vi "NOPTR_Mem_DataToU8Array.vi"(8 "error in (no error)":errorcluster, 10 "Payload":variant, 11 "AddrQueueIn":refnum<queue>) -> (0 "error out":errorcluster, 1 "Supported Type?":bool, 2 "ByteArray":u8[](array[numeric]), 3 "AddrQueueOut":refnum<queue>)   [LabVIEW 2019, in "Memory Data Access.lvlib"]
uses:
  Memory Data Access.lvlib
  <vilib>/Utility/Data Type/Type Definitions/Data Type.ctl
  Global/Global.vi
  <vilib>/Utility/Data Type/NI_Data Type.lvlib
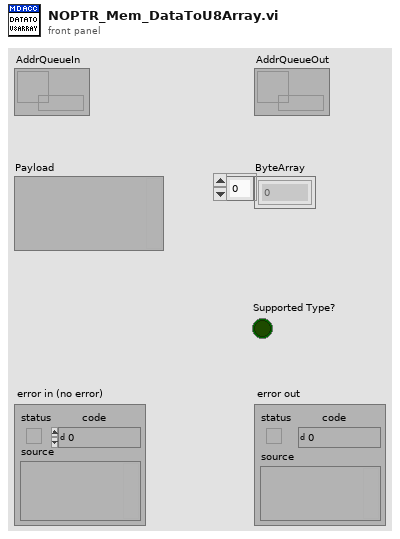
[diagram p1: front panel]
types:
  T1 = typedef "NI_Data Type.lvlib/Data Type.ctl" = enum8{"Invalid Type", "Void", "I8", "I16", "I32", "I64", "U8", "U16", "U32", "U64", "Single Float", "Double Float", "Extended Float", "Single Complex", "Double Complex", "Extended Complex", "Enum U8", "Enum U16", "Enum U32", "Enum U64", "Single Float With Unit", "Double Float With Unit", "Extended Float With Unit", "Single Complex with Unit", "Double Complex with Unit", "Extended Complex with Unit", "Boolean", "String", "Path", "Picture", "Tag", "Array", "Cluster", "Variant", "LV Variant", "Waveform", "Timestamp", "Digital Waveform", "Digital Data", "ExpressData", "Refnum", "External Data", "VI", "Poly VI", "LabVIEW Class Instance", "Fixed Point", "Set Collection", "Map Collection"}
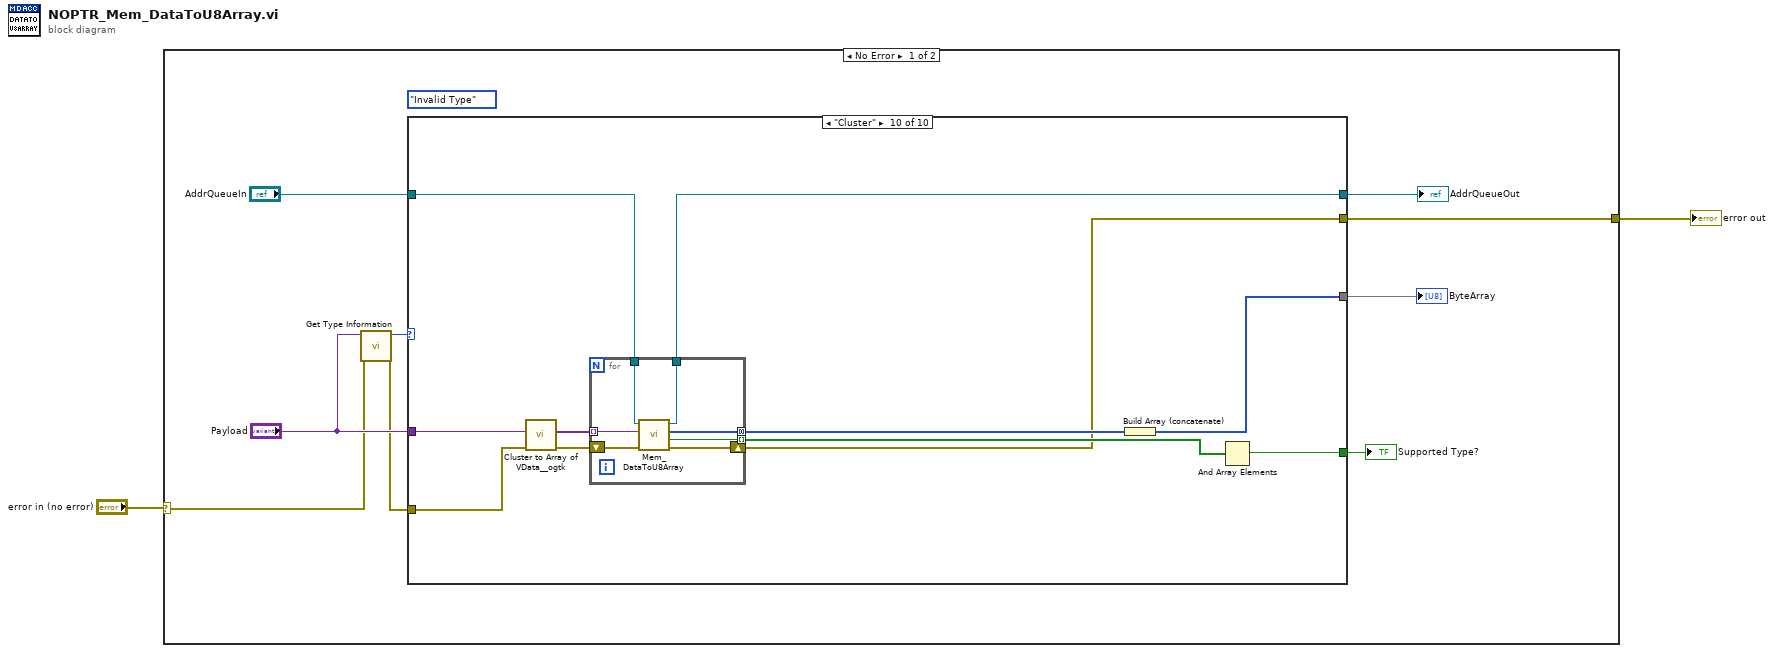
[diagram p0: block diagram]
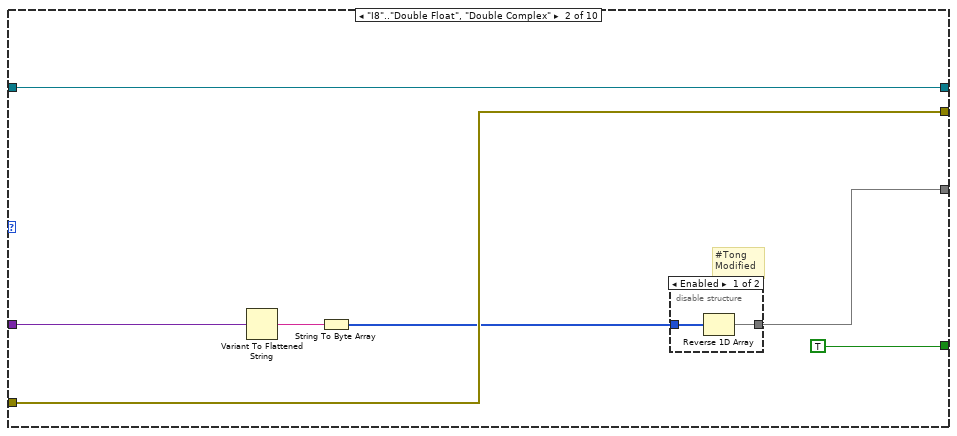
[diagram p3: hidden frame]
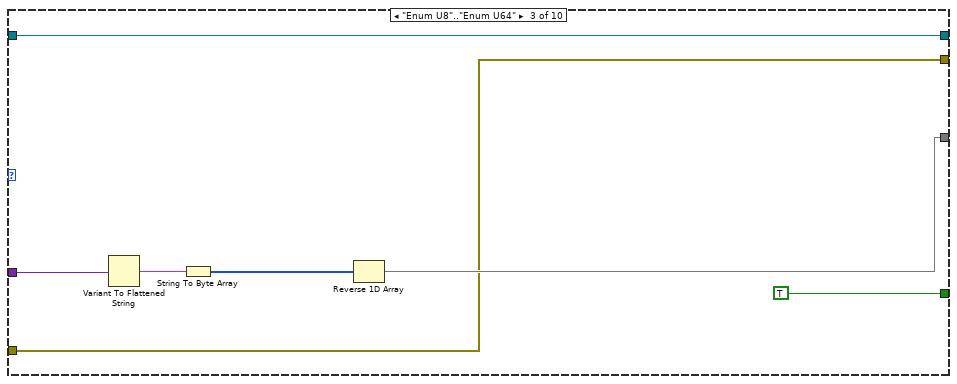
[diagram p5: hidden frame]
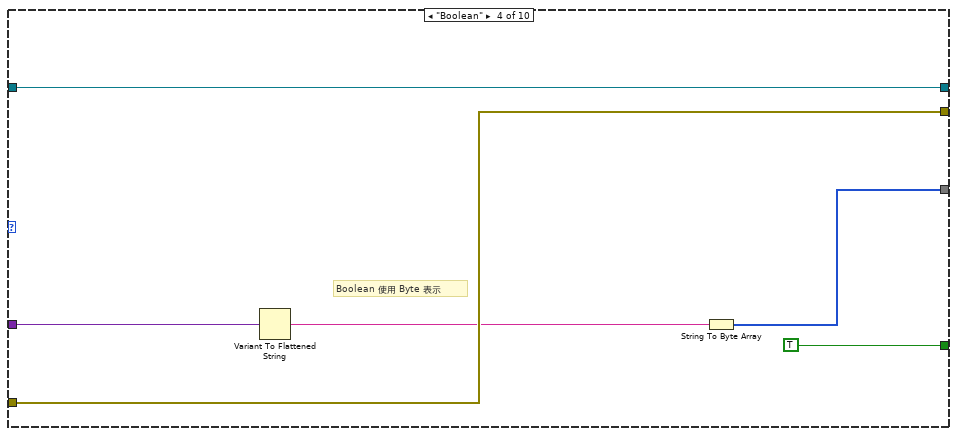
[diagram p6: hidden frame]
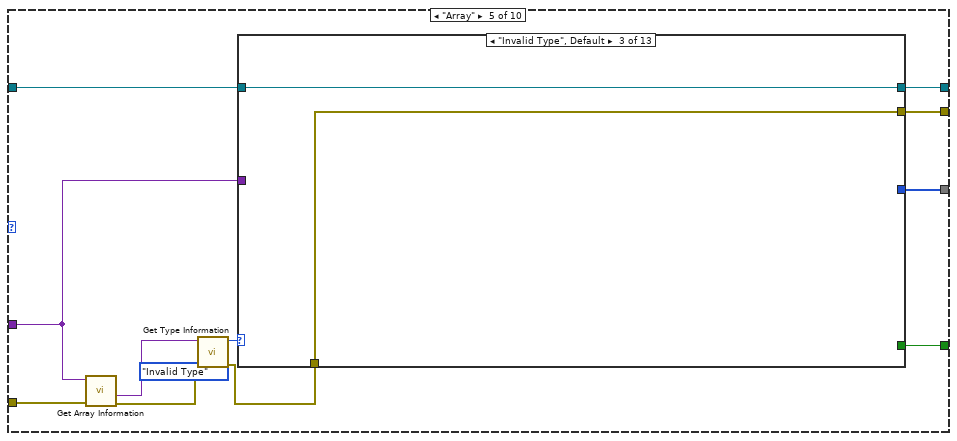
[diagram p7: hidden frame]
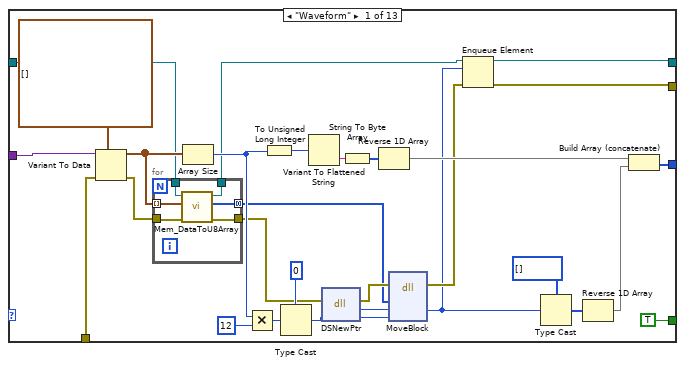
[diagram p8: hidden frame]
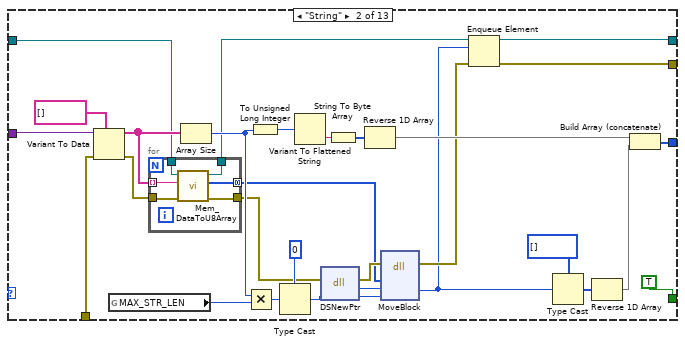
[diagram p9: hidden frame]
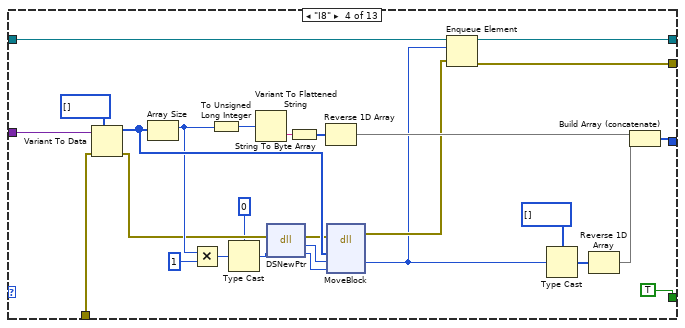
[diagram p10: hidden frame]
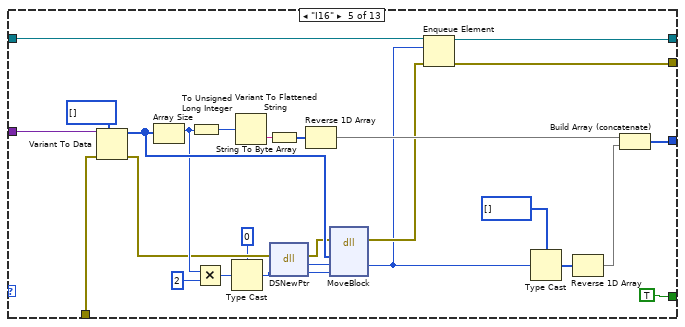
[diagram p11: hidden frame]
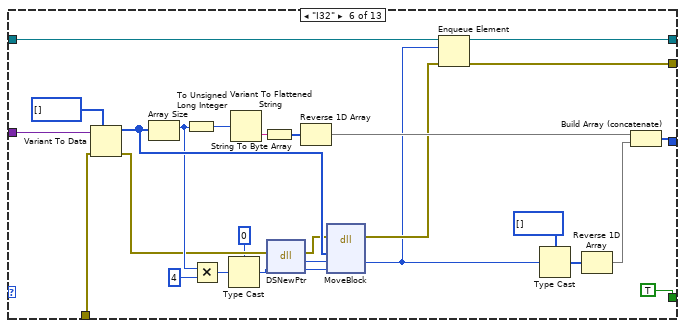
[diagram p12: hidden frame]
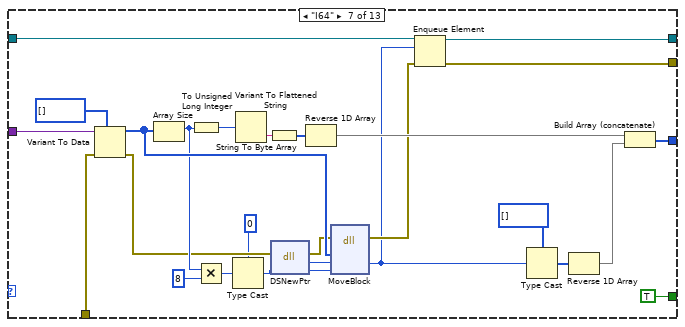
[diagram p13: hidden frame]
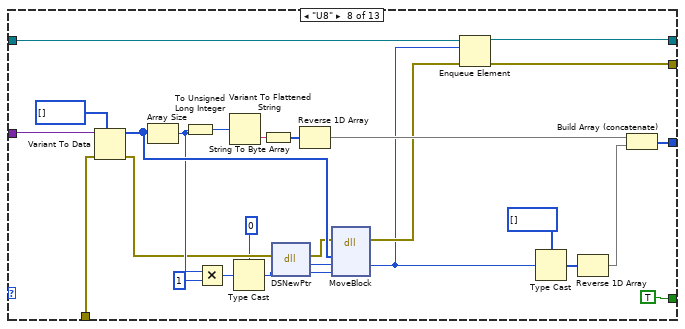
[diagram p14: hidden frame]
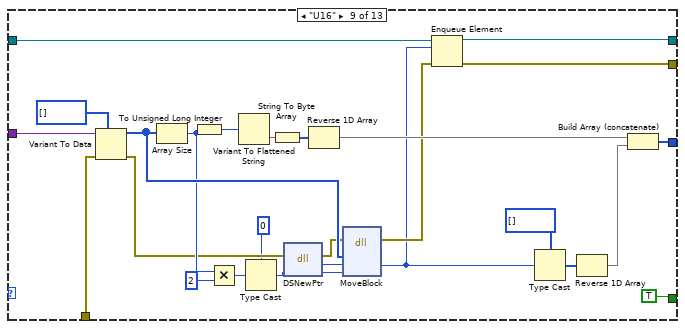
[diagram p15: hidden frame]
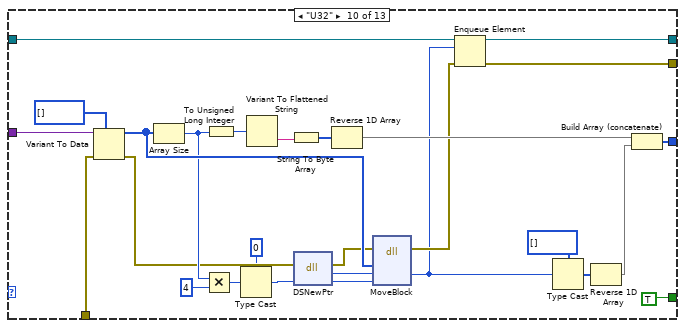
[diagram p16: hidden frame]
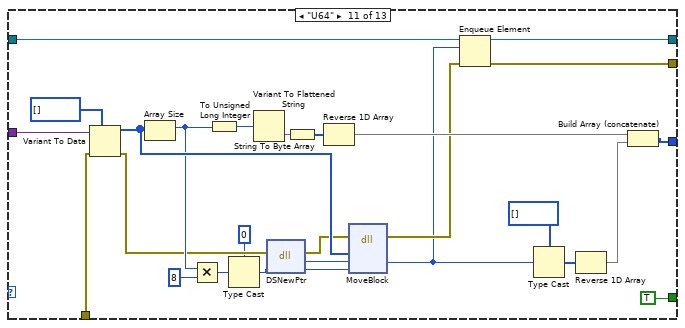
[diagram p17: hidden frame]
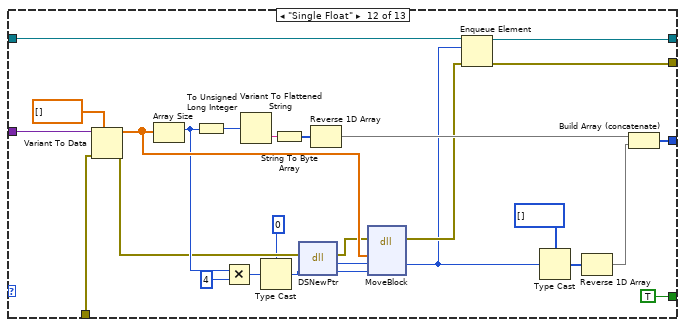
[diagram p18: hidden frame]
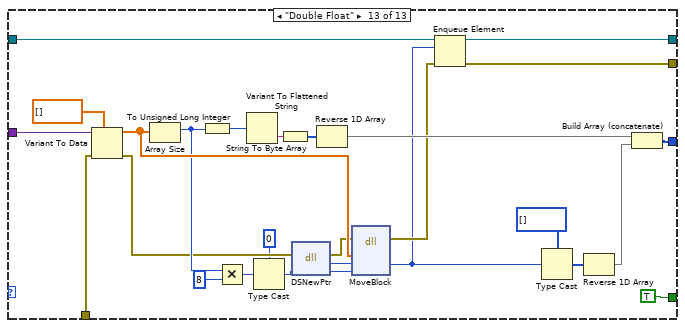
[diagram p19: hidden frame]
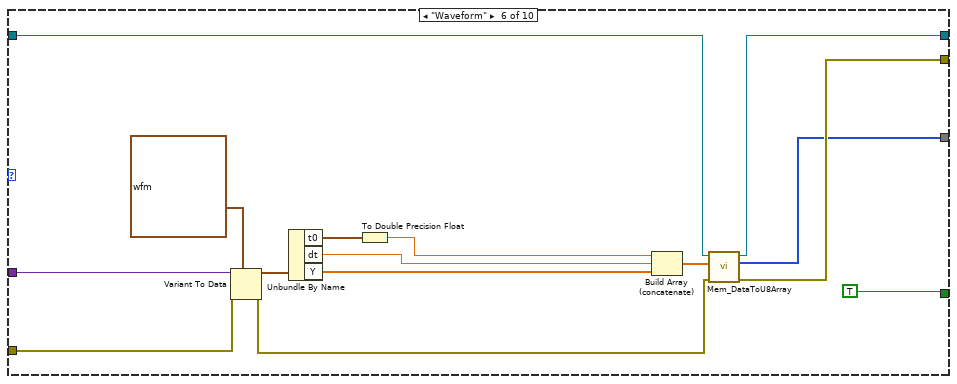
[diagram p20: hidden frame]
diagram:
  n1 = case shown="No Error" "error in (no error)" {
    selector: "error in (no error)" -> [w3 w466]
    tunnel: [w11 w466] -> w2
    frame No Error {
      (unwired) Data_Type."Invalid Type" ("Type")
      n2 = call <vilib>:"Get Type Information.vi"("error in (no error)"=w3, "variant"="Payload") -> ("error out"=w6:errorcluster, "type"=w7:T1)  [unwired: 5 in, 3 out]
      n3 = case shown="\"Cluster\"" w7 {
        tunnel: w6 -> [w13 w20 w26 w36 w44 w398 w409 w429 w438 w450]
        tunnel: [w13 w20 w26 w36 w46 w395 w410 w430 w439 w451] -> w11
        tunnel: [_ w15 w27 w32 w47 w394 w412 w425 w441 w455] -> w10
        tunnel: "Payload" -> [_ w18 w29 w34 w45 w405 w413 w433 w442 w458]
        tunnel: [_ TRUE TRUE ("Supported Type?") TRUE w37 TRUE TRUE TRUE TRUE w453] -> w9
        tunnel: "AddrQueueIn" -> [w12 w14 w24 w31 w40 w393 w407 w424 w435 w449]
        tunnel: [w12 w14 w24 w31 w39 w392 w407 w424 w435 w448] -> w4
        frame "Invalid Type", Default {
        }
        frame "I8".."Double Float", "Double Complex" {
          # "#Tong\nModified"
          n4 = Variant To Flattened String(Variant=w18) -> (data string=w17:string)  [unwired: 1 out]
          n5 = String To Byte Array(string=w17) -> (unsigned byte array=w16:u8[])
          n6 = disable-structure shown="Enabled" {
            disable-tunnel: w16 -> [w22 w23]
            disable-tunnel: [w21 w23] -> w15
            frame Enabled {
              n7 = Reverse 1D Array(array=w22) -> (reversed array=w21:u8[])
            }
            frame Disabled {
            }
          }
        }
        frame "Enum U8".."Enum U64" {
          n8 = Variant To Flattened String(Variant=w29) -> (data string=w30:string)  [unwired: 1 out]
          n9 = String To Byte Array(string=w30) -> (unsigned byte array=w28:u8[])
          n10 = Reverse 1D Array(array=w28) -> (reversed array=w27:u8[])
        }
        frame "Boolean" {
          # "Boolean 使用 Byte 表示"
          n11 = Variant To Flattened String(Variant=w34) -> (data string=w33:string)  [unwired: 1 out]
          n12 = String To Byte Array(string=w33) -> (unsigned byte array=w32:u8[])
        }
        frame "Array" {
          (unwired) Data_Type."Invalid Type" ("type")
          n13 = call <vilib>:"Get Array Information.vi"("error in (no error)"=w44, "variant"=w45) -> ("error out"=w38:errorcluster, "array element data type"=w42:variant)  [unwired: 6 in, 2 out]
          n14 = call <vilib>:"Get Type Information.vi"("error in (no error)"=w38, "variant"=w42) -> ("error out"=w41:errorcluster, "type"=w43:T1)  [unwired: 5 in, 3 out]
          n15 = case shown="\"Invalid Type\", Default" w43 {
            tunnel: [w58 w97 _ w128 w156 w183 w210 w236 w263 w290 w317 w344 w371] -> w47
            tunnel: w45 -> [w57 w98 _ w130 w157 w184 w211 w238 w265 w293 w319 w346 w373]
            tunnel: w41 -> [w56 w96 w120 w129 w155 w182 w209 w237 w264 w292 w318 w345 w372]
            tunnel: [w51 w88 w120 w124 w152 w178 w204 w231 w259 w287 w313 w340 w368] -> w46
            tunnel: w40 -> [w50 w87 w121 w127 w154 w181 w208 w235 w262 w289 w316 w343 w370]
            tunnel: [w55 w90 w121 w126 w153 w180 w207 w234 w261 w285 w315 w342 w367] -> w39
            tunnel: [TRUE ("Supported Type?") TRUE ("Supported Type?") _ TRUE ("Supported Type?") TRUE ("Supported Type?") TRUE ("Supported Type?") TRUE ("Supported Type?") TRUE ("Supported Type?") TRUE ("Supported Type?") TRUE ("Supported Type?") TRUE ("Supported Type?") TRUE ("Supported Type?") TRUE ("Supported Type?")] -> w37
            frame "Waveform" {
              n16 = Variant To Data(error in=w56, type=waveform(dbl)[] [], Variant=w57) -> (data=w62:waveform(dbl)[], error out=w61:errorcluster)
              n17 = for {
                tunnel: w62 -> [w83] mode=indexing
                tunnel: w61 -> [w82]
                tunnel: [w81] -> w59 mode=concatenating
                tunnel: [w80] -> w60
                tunnel: w50 -> [w79]
                tunnel: [w78] -> w49
                n18 = call "Mem_DataToU8Array.vi"("error in (no error)"=w82, "Payload"=w83, "AddrQueueIn"=w79) -> ("error out"=w80:errorcluster, "ByteArray"=w81:u8[], "AddrQueueOut"=w78:refnum<queue>)  [unwired: 5 in, 1 out]
              }
              n19 = Array Size(array=w62) -> (size(s)=w73:i32)
              n20 = Multiply(x=w73, y=12) -> (x*y=w74:i32)
              n21 = To Unsigned Long Integer(number=w73) -> (unsigned 32bit integer=w70:u32)
              n22 = Type Cast(type=u32 0, x=w74) -> (*(type *) &x=w75:u32)
              n23 = Variant To Flattened String(Variant=w70) -> (data string=w69:string)  [unwired: 1 out]
              n24 = dll-call lib="LabVIEW" fn="DSNewPtr"(error in=w60, "size"=w75) -> (error out=w66:errorcluster, "return type"=w76:u64, "size"=w77:u32)  [unwired: 2 in, 1 out]
              n25 = String To Byte Array(string=w69) -> (unsigned byte array=w71:u8[])
              n26 = Reverse 1D Array(array=w71) -> (reversed array=w72:u8[])
              n27 = dll-call lib="LabVIEW" fn="MoveBlock"(error in=w66, "PointerSRC"=w59, "PointerDEST"=w76, "size"=w77) -> (error out=w53:errorcluster, "PointerDEST"=w52:u64)  [unwired: 5 in, 1 out]
              n28 = Enqueue Element(queue=w49, element=w52, error in (no error)=w53) -> (queue out=w55:refnum<queue>, error out=w51:errorcluster)  [unwired: 1 in, 1 out]
              n29 = Type Cast(type=u8[] [], x=w52) -> (*(type *) &x=w68:u8[])
              n30 = Reverse 1D Array(array=w68) -> (reversed array=w67:u8[])
              n31 = Build Array (concatenate)(w72, w67) -> (w58:u8[])
            }
            frame "String" {
              n32 = Variant To Data(error in=w96, type=string[] [], Variant=w98) -> (data=w95:string[], error out=w94:errorcluster)
              n33 = global read "Global.vi" "MAX_STR_LEN"() -> (w91:u32)
              n34 = for {
                tunnel: w95 -> [w119] mode=indexing
                tunnel: w94 -> [w118]
                tunnel: [w117] -> w92 mode=concatenating
                tunnel: [w116] -> w93
                tunnel: w87 -> [w115]
                tunnel: [w114] -> w85
                n35 = call "Mem_DataToU8Array.vi"("error in (no error)"=w118, "Payload"=w119, "AddrQueueIn"=w115) -> ("error out"=w116:errorcluster, "ByteArray"=w117:u8[], "AddrQueueOut"=w114:refnum<queue>)  [unwired: 5 in, 1 out]
              }
              n36 = Array Size(array=w95) -> (size(s)=w109:i32)
              n37 = Multiply(x=w109, y=w91) -> (x*y=w110:u32)
              n38 = To Unsigned Long Integer(number=w109) -> (unsigned 32bit integer=w106:u32)
              n39 = Type Cast(type=u32 0, x=w110) -> (*(type *) &x=w111:u32)
              n40 = Variant To Flattened String(Variant=w106) -> (data string=w105:string)  [unwired: 1 out]
              n41 = dll-call lib="LabVIEW" fn="DSNewPtr"(error in=w93, "size"=w111) -> (error out=w102:errorcluster, "return type"=w112:u64, "size"=w113:u32)  [unwired: 2 in, 1 out]
              n42 = String To Byte Array(string=w105) -> (unsigned byte array=w107:u8[])
              n43 = Reverse 1D Array(array=w107) -> (reversed array=w108:u8[])
              n44 = dll-call lib="LabVIEW" fn="MoveBlock"(error in=w102, "PointerSRC"=w92, "PointerDEST"=w112, "size"=w113) -> (error out=w89:errorcluster, "PointerDEST"=w86:u64)  [unwired: 5 in, 1 out]
              n45 = Enqueue Element(queue=w85, element=w86, error in (no error)=w89) -> (queue out=w90:refnum<queue>, error out=w88:errorcluster)  [unwired: 1 in, 1 out]
              n46 = Type Cast(type=u8[] [], x=w86) -> (*(type *) &x=w104:u8[])
              n47 = Reverse 1D Array(array=w104) -> (reversed array=w103:u8[])
              n48 = Build Array (concatenate)(w108, w103) -> (w97:u8[])
            }
            frame "Invalid Type", Default {
            }
            frame "I8" {
              n49 = Variant To Data(error in=w129, type=i8[] [], Variant=w130) -> (data=w146:i8[], error out=w138:errorcluster)
              n50 = Array Size(array=w146) -> (size(s)=w143:i32)
              n51 = Multiply(x=w143, y=1) -> (x*y=w144:i32)
              n52 = To Unsigned Long Integer(number=w143) -> (unsigned 32bit integer=w140:u32)
              n53 = Type Cast(type=u32 0, x=w144) -> (*(type *) &x=w145:u32)
              n54 = Variant To Flattened String(Variant=w140) -> (data string=w139:string)  [unwired: 1 out]
              n55 = dll-call lib="LabVIEW" fn="DSNewPtr"(error in=w138, "size"=w145) -> (error out=w135:errorcluster, "return type"=w147:u64, "size"=w148:u32)  [unwired: 2 in, 1 out]
              n56 = String To Byte Array(string=w139) -> (unsigned byte array=w141:u8[])
              n57 = Reverse 1D Array(array=w141) -> (reversed array=w142:u8[])
              n58 = dll-call lib="LabVIEW" fn="MoveBlock"(error in=w135, "PointerSRC"=w146, "PointerDEST"=w147, "size"=w148) -> (error out=w125:errorcluster, "PointerDEST"=w123:u64)  [unwired: 5 in, 1 out]
              n59 = Enqueue Element(queue=w127, element=w123, error in (no error)=w125) -> (queue out=w126:refnum<queue>, error out=w124:errorcluster)  [unwired: 1 in, 1 out]
              n60 = Type Cast(type=u8[] [], x=w123) -> (*(type *) &x=w137:u8[])
              n61 = Reverse 1D Array(array=w137) -> (reversed array=w136:u8[])
              n62 = Build Array (concatenate)(w142, w136) -> (w128:u8[])
            }
            frame "I16" {
              n63 = Variant To Data(error in=w155, type=i16[] [], Variant=w157) -> (data=w173:i16[], error out=w165:errorcluster)
              n64 = Array Size(array=w173) -> (size(s)=w170:i32)
              n65 = To Unsigned Long Integer(number=w170) -> (unsigned 32bit integer=w167:u32)
              n66 = Multiply(x=w170, y=2) -> (x*y=w171:i32)
              n67 = Type Cast(type=u32 0, x=w171) -> (*(type *) &x=w172:u32)
              n68 = Variant To Flattened String(Variant=w167) -> (data string=w166:string)  [unwired: 1 out]
              n69 = String To Byte Array(string=w166) -> (unsigned byte array=w168:u8[])
              n70 = dll-call lib="LabVIEW" fn="DSNewPtr"(error in=w165, "size"=w172) -> (error out=w162:errorcluster, "return type"=w174:u64, "size"=w175:u32)  [unwired: 2 in, 1 out]
              n71 = Reverse 1D Array(array=w168) -> (reversed array=w169:u8[])
              n72 = dll-call lib="LabVIEW" fn="MoveBlock"(error in=w162, "PointerSRC"=w173, "PointerDEST"=w174, "size"=w175) -> (error out=w151:errorcluster, "PointerDEST"=w150:u64)  [unwired: 5 in, 1 out]
              n73 = Enqueue Element(queue=w154, element=w150, error in (no error)=w151) -> (queue out=w153:refnum<queue>, error out=w152:errorcluster)  [unwired: 1 in, 1 out]
              n74 = Type Cast(type=u8[] [], x=w150) -> (*(type *) &x=w164:u8[])
              n75 = Reverse 1D Array(array=w164) -> (reversed array=w163:u8[])
              n76 = Build Array (concatenate)(w169, w163) -> (w156:u8[])
            }
            frame "I32" {
              n77 = Variant To Data(error in=w182, type=i32[] [], Variant=w184) -> (data=w200:i32[], error out=w192:errorcluster)
              n78 = Array Size(array=w200) -> (size(s)=w197:i32)
              n79 = To Unsigned Long Integer(number=w197) -> (unsigned 32bit integer=w194:u32)
              n80 = Multiply(x=w197, y=4) -> (x*y=w198:i32)
              n81 = Type Cast(type=u32 0, x=w198) -> (*(type *) &x=w199:u32)
              n82 = Variant To Flattened String(Variant=w194) -> (data string=w193:string)  [unwired: 1 out]
              n83 = String To Byte Array(string=w193) -> (unsigned byte array=w195:u8[])
              n84 = dll-call lib="LabVIEW" fn="DSNewPtr"(error in=w192, "size"=w199) -> (error out=w189:errorcluster, "return type"=w201:u64, "size"=w202:u32)  [unwired: 2 in, 1 out]
              n85 = Reverse 1D Array(array=w195) -> (reversed array=w196:u8[])
              n86 = dll-call lib="LabVIEW" fn="MoveBlock"(error in=w189, "PointerSRC"=w200, "PointerDEST"=w201, "size"=w202) -> (error out=w179:errorcluster, "PointerDEST"=w177:u64)  [unwired: 5 in, 1 out]
              n87 = Enqueue Element(queue=w181, element=w177, error in (no error)=w179) -> (queue out=w180:refnum<queue>, error out=w178:errorcluster)  [unwired: 1 in, 1 out]
              n88 = Type Cast(type=u8[] [], x=w177) -> (*(type *) &x=w191:u8[])
              n89 = Reverse 1D Array(array=w191) -> (reversed array=w190:u8[])
              n90 = Build Array (concatenate)(w196, w190) -> (w183:u8[])
            }
            frame "I64" {
              n91 = Variant To Data(error in=w209, type=i64[] [], Variant=w211) -> (data=w227:i64[], error out=w219:errorcluster)
              n92 = Array Size(array=w227) -> (size(s)=w224:i32)
              n93 = To Unsigned Long Integer(number=w224) -> (unsigned 32bit integer=w221:u32)
              n94 = Multiply(x=w224, y=8) -> (x*y=w225:i32)
              n95 = Type Cast(type=u32 0, x=w225) -> (*(type *) &x=w226:u32)
              n96 = Variant To Flattened String(Variant=w221) -> (data string=w220:string)  [unwired: 1 out]
              n97 = String To Byte Array(string=w220) -> (unsigned byte array=w222:u8[])
              n98 = dll-call lib="LabVIEW" fn="DSNewPtr"(error in=w219, "size"=w226) -> (error out=w216:errorcluster, "return type"=w228:u64, "size"=w229:u32)  [unwired: 2 in, 1 out]
              n99 = Reverse 1D Array(array=w222) -> (reversed array=w223:u8[])
              n100 = dll-call lib="LabVIEW" fn="MoveBlock"(error in=w216, "PointerSRC"=w227, "PointerDEST"=w228, "size"=w229) -> (error out=w206:errorcluster, "PointerDEST"=w205:u64)  [unwired: 5 in, 1 out]
              n101 = Enqueue Element(queue=w208, element=w205, error in (no error)=w206) -> (queue out=w207:refnum<queue>, error out=w204:errorcluster)  [unwired: 1 in, 1 out]
              n102 = Type Cast(type=u8[] [], x=w205) -> (*(type *) &x=w218:u8[])
              n103 = Reverse 1D Array(array=w218) -> (reversed array=w217:u8[])
              n104 = Build Array (concatenate)(w223, w217) -> (w210:u8[])
            }
            frame "U8" {
              n105 = Variant To Data(error in=w237, type=u8[] [], Variant=w238) -> (data=w254:u8[], error out=w246:errorcluster)
              n106 = Array Size(array=w254) -> (size(s)=w251:i32)
              n107 = To Unsigned Long Integer(number=w251) -> (unsigned 32bit integer=w248:u32)
              n108 = Multiply(x=w251, y=1) -> (x*y=w252:i32)
              n109 = Variant To Flattened String(Variant=w248) -> (data string=w247:string)  [unwired: 1 out]
              n110 = Type Cast(type=u32 0, x=w252) -> (*(type *) &x=w253:u32)
              n111 = String To Byte Array(string=w247) -> (unsigned byte array=w249:u8[])
              n112 = dll-call lib="LabVIEW" fn="DSNewPtr"(error in=w246, "size"=w253) -> (error out=w243:errorcluster, "return type"=w255:u64, "size"=w256:u32)  [unwired: 2 in, 1 out]
              n113 = Reverse 1D Array(array=w249) -> (reversed array=w250:u8[])
              n114 = dll-call lib="LabVIEW" fn="MoveBlock"(error in=w243, "PointerSRC"=w254, "PointerDEST"=w255, "size"=w256) -> (error out=w233:errorcluster, "PointerDEST"=w232:u64)  [unwired: 5 in, 1 out]
              n115 = Enqueue Element(queue=w235, element=w232, error in (no error)=w233) -> (queue out=w234:refnum<queue>, error out=w231:errorcluster)  [unwired: 1 in, 1 out]
              n116 = Type Cast(type=u8[] [], x=w232) -> (*(type *) &x=w245:u8[])
              n117 = Reverse 1D Array(array=w245) -> (reversed array=w244:u8[])
              n118 = Build Array (concatenate)(w250, w244) -> (w236:u8[])
            }
            frame "U16" {
              n119 = Variant To Data(error in=w264, type=u16[] [], Variant=w265) -> (data=w281:u16[], error out=w273:errorcluster)
              n120 = Array Size(array=w281) -> (size(s)=w278:i32)
              n121 = To Unsigned Long Integer(number=w278) -> (unsigned 32bit integer=w275:u32)
              n122 = Multiply(x=w278, y=2) -> (x*y=w279:i32)
              n123 = Variant To Flattened String(Variant=w275) -> (data string=w274:string)  [unwired: 1 out]
              n124 = Type Cast(type=u32 0, x=w279) -> (*(type *) &x=w280:u32)
              n125 = String To Byte Array(string=w274) -> (unsigned byte array=w276:u8[])
              n126 = dll-call lib="LabVIEW" fn="DSNewPtr"(error in=w273, "size"=w280) -> (error out=w270:errorcluster, "return type"=w282:u64, "size"=w283:u32)  [unwired: 2 in, 1 out]
              n127 = Reverse 1D Array(array=w276) -> (reversed array=w277:u8[])
              n128 = dll-call lib="LabVIEW" fn="MoveBlock"(error in=w270, "PointerSRC"=w281, "PointerDEST"=w282, "size"=w283) -> (error out=w260:errorcluster, "PointerDEST"=w258:u64)  [unwired: 5 in, 1 out]
              n129 = Enqueue Element(queue=w262, element=w258, error in (no error)=w260) -> (queue out=w261:refnum<queue>, error out=w259:errorcluster)  [unwired: 1 in, 1 out]
              n130 = Type Cast(type=u8[] [], x=w258) -> (*(type *) &x=w272:u8[])
              n131 = Reverse 1D Array(array=w272) -> (reversed array=w271:u8[])
              n132 = Build Array (concatenate)(w277, w271) -> (w263:u8[])
            }
            frame "U32" {
              n133 = Variant To Data(error in=w292, type=u32[] [], Variant=w293) -> (data=w308:u32[], error out=w300:errorcluster)
              n134 = Array Size(array=w308) -> (size(s)=w305:i32)
              n135 = Multiply(x=w305, y=4) -> (x*y=w306:i32)
              n136 = To Unsigned Long Integer(number=w305) -> (unsigned 32bit integer=w302:u32)
              n137 = Type Cast(type=u32 0, x=w306) -> (*(type *) &x=w307:u32)
              n138 = Variant To Flattened String(Variant=w302) -> (data string=w301:string)  [unwired: 1 out]
              n139 = String To Byte Array(string=w301) -> (unsigned byte array=w303:u8[])
              n140 = dll-call lib="LabVIEW" fn="DSNewPtr"(error in=w300, "size"=w307) -> (error out=w297:errorcluster, "return type"=w309:u64, "size"=w310:u32)  [unwired: 2 in, 1 out]
              n141 = Reverse 1D Array(array=w303) -> (reversed array=w304:u8[])
              n142 = dll-call lib="LabVIEW" fn="MoveBlock"(error in=w297, "PointerSRC"=w308, "PointerDEST"=w309, "size"=w310) -> (error out=w288:errorcluster, "PointerDEST"=w286:u64)  [unwired: 5 in, 1 out]
              n143 = Enqueue Element(queue=w289, element=w286, error in (no error)=w288) -> (queue out=w285:refnum<queue>, error out=w287:errorcluster)  [unwired: 1 in, 1 out]
              n144 = Type Cast(type=u8[] [], x=w286) -> (*(type *) &x=w299:u8[])
              n145 = Reverse 1D Array(array=w299) -> (reversed array=w298:u8[])
              n146 = Build Array (concatenate)(w304, w298) -> (w290:u8[])
            }
            frame "U64" {
              n147 = Variant To Data(error in=w318, type=u64[] [], Variant=w319) -> (data=w335:u64[], error out=w327:errorcluster)
              n148 = Array Size(array=w335) -> (size(s)=w332:i32)
              n149 = Multiply(x=w332, y=8) -> (x*y=w333:i32)
              n150 = To Unsigned Long Integer(number=w332) -> (unsigned 32bit integer=w329:u32)
              n151 = Type Cast(type=u32 0, x=w333) -> (*(type *) &x=w334:u32)
              n152 = Variant To Flattened String(Variant=w329) -> (data string=w328:string)  [unwired: 1 out]
              n153 = dll-call lib="LabVIEW" fn="DSNewPtr"(error in=w327, "size"=w334) -> (error out=w324:errorcluster, "return type"=w336:u64, "size"=w337:u32)  [unwired: 2 in, 1 out]
              n154 = String To Byte Array(string=w328) -> (unsigned byte array=w330:u8[])
              n155 = Reverse 1D Array(array=w330) -> (reversed array=w331:u8[])
              n156 = dll-call lib="LabVIEW" fn="MoveBlock"(error in=w324, "PointerSRC"=w335, "PointerDEST"=w336, "size"=w337) -> (error out=w314:errorcluster, "PointerDEST"=w312:u64)  [unwired: 5 in, 1 out]
              n157 = Enqueue Element(queue=w316, element=w312, error in (no error)=w314) -> (queue out=w315:refnum<queue>, error out=w313:errorcluster)  [unwired: 1 in, 1 out]
              n158 = Type Cast(type=u8[] [], x=w312) -> (*(type *) &x=w326:u8[])
              n159 = Reverse 1D Array(array=w326) -> (reversed array=w325:u8[])
              n160 = Build Array (concatenate)(w331, w325) -> (w317:u8[])
            }
            frame "Single Float" {
              n161 = Variant To Data(error in=w345, type=sgl[] [], Variant=w346) -> (data=w362:sgl[], error out=w354:errorcluster)
              n162 = Array Size(array=w362) -> (size(s)=w359:i32)
              n163 = To Unsigned Long Integer(number=w359) -> (unsigned 32bit integer=w356:u32)
              n164 = Multiply(x=w359, y=4) -> (x*y=w360:i32)
              n165 = Variant To Flattened String(Variant=w356) -> (data string=w355:string)  [unwired: 1 out]
              n166 = Type Cast(type=u32 0, x=w360) -> (*(type *) &x=w361:u32)
              n167 = String To Byte Array(string=w355) -> (unsigned byte array=w357:u8[])
              n168 = dll-call lib="LabVIEW" fn="DSNewPtr"(error in=w354, "size"=w361) -> (error out=w351:errorcluster, "return type"=w363:u64, "size"=w364:u32)  [unwired: 2 in, 1 out]
              n169 = Reverse 1D Array(array=w357) -> (reversed array=w358:u8[])
              n170 = dll-call lib="LabVIEW" fn="MoveBlock"(error in=w351, "PointerSRC"=w362, "PointerDEST"=w363, "size"=w364) -> (error out=w341:errorcluster, "PointerDEST"=w339:u64)  [unwired: 5 in, 1 out]
              n171 = Enqueue Element(queue=w343, element=w339, error in (no error)=w341) -> (queue out=w342:refnum<queue>, error out=w340:errorcluster)  [unwired: 1 in, 1 out]
              n172 = Type Cast(type=u8[] [], x=w339) -> (*(type *) &x=w353:u8[])
              n173 = Reverse 1D Array(array=w353) -> (reversed array=w352:u8[])
              n174 = Build Array (concatenate)(w358, w352) -> (w344:u8[])
            }
            frame "Double Float" {
              n175 = Variant To Data(error in=w372, type=dbl[] [], Variant=w373) -> (data=w389:dbl[], error out=w381:errorcluster)
              n176 = Array Size(array=w389) -> (size(s)=w386:i32)
              n177 = To Unsigned Long Integer(number=w386) -> (unsigned 32bit integer=w383:u32)
              n178 = Multiply(x=w386, y=8) -> (x*y=w387:i32)
              n179 = Variant To Flattened String(Variant=w383) -> (data string=w382:string)  [unwired: 1 out]
              n180 = Type Cast(type=u32 0, x=w387) -> (*(type *) &x=w388:u32)
              n181 = String To Byte Array(string=w382) -> (unsigned byte array=w384:u8[])
              n182 = dll-call lib="LabVIEW" fn="DSNewPtr"(error in=w381, "size"=w388) -> (error out=w378:errorcluster, "return type"=w390:u64, "size"=w391:u32)  [unwired: 2 in, 1 out]
              n183 = Reverse 1D Array(array=w384) -> (reversed array=w385:u8[])
              n184 = dll-call lib="LabVIEW" fn="MoveBlock"(error in=w378, "PointerSRC"=w389, "PointerDEST"=w390, "size"=w391) -> (error out=w369:errorcluster, "PointerDEST"=w366:u64)  [unwired: 5 in, 1 out]
              n185 = Enqueue Element(queue=w370, element=w366, error in (no error)=w369) -> (queue out=w367:refnum<queue>, error out=w368:errorcluster)  [unwired: 1 in, 1 out]
              n186 = Type Cast(type=u8[] [], x=w366) -> (*(type *) &x=w380:u8[])
              n187 = Reverse 1D Array(array=w380) -> (reversed array=w379:u8[])
              n188 = Build Array (concatenate)(w385, w379) -> (w371:u8[])
            }
          }
        }
        frame "Waveform" {
          n189 = Variant To Data(error in=w398, type=waveform(dbl) {"t0"=timestamp(0 s since 1904-01-01), "dt"=1.0, "Y"=[]} ("Waveform"), Variant=w405) -> (data=w403:waveform(dbl), error out=w396:errorcluster)
          n190 = Unbundle By Name(w403) -> ("t0"=w401:timestamp, "dt"=w399:dbl, "Y"=w402:dbl[])
          n191 = To Double Precision Float(number=w401) -> (double precision float=w400:dbl)
          n192 = Build Array (concatenate)(w400, w399, w402) -> (w397:dbl[])
          n193 = call "Mem_DataToU8Array.vi"("error in (no error)"=w396, "Payload"=w397, "AddrQueueIn"=w393) -> ("error out"=w395:errorcluster, "ByteArray"=w394:u8[], "AddrQueueOut"=w392:refnum<queue>)  [unwired: 5 in, 1 out]
        }
        frame "String" {
          # "#Tong\nmodified"
          n194 = Variant To Data(error in=w409, type="" ("Waveform"), Variant=w413) -> (data=w408:string, error out=w410:errorcluster)
          n195 = disable-structure shown="Enabled" {
            disable-tunnel: [w417 w419] -> w412
            disable-tunnel: w408 -> [w416 w421]
            frame Disabled {
              n196 = String To Byte Array(string=w416) -> (unsigned byte array=w415:u8[])
              n197 = Variant To Flattened String(Variant=w415) -> (data string=w417:string)  [unwired: 1 out]
            }
            frame Enabled {
              n198 = global read "Global.vi" "MAX_STR_LEN"() -> (w418:u32)
              n199 = String To Byte Array(string=w421) -> (unsigned byte array=w420:u8[])
              n200 = Initialize Array(u8 0 ("*(type *) &x"), w418) -> (w422:u8[])
              n201 = Replace Array Subset(array=w422, new element=w420) -> (w419:u8[])  [unwired: 1 in]
            }
          }
        }
        frame "Timestamp" {
          n202 = Variant To Data(error in=w429, type=timestamp(0 s since 1904-01-01) ("Waveform"), Variant=w433) -> (data=w428:timestamp, error out=w430:errorcluster)
          n203 = To Double Precision Float(number=w428) -> (double precision float=w427:dbl)
          n204 = Variant To Flattened String(Variant=w427) -> (data string=w432:string)  [unwired: 1 out]
          n205 = String To Byte Array(string=w432) -> (unsigned byte array=w426:u8[])
          n206 = Reverse 1D Array(array=w426) -> (reversed array=w425:u8[])
        }
        frame "Path" {
          n207 = Variant To Data(error in=w438, type=path "" ("Waveform"), Variant=w442) -> (data=w437:path, error out=w439:errorcluster)
          n208 = Path To String(path=w437) -> (string=w436:string)
          n209 = disable-structure shown="Enabled" {
            disable-tunnel: [w445 w446] -> w441
            disable-tunnel: w436 -> [w444 w447]
            frame Disabled {
              n210 = Variant To Flattened String(Variant=w444) -> (data string=w445:string)  [unwired: 1 out]
            }
            frame Enabled {
              n211 = String To Byte Array(string=w447) -> (unsigned byte array=w446:u8[])
            }
          }
        }
        frame "Cluster" {
          n212 = call <userlib>:"Cluster to Array of VData__ogtk.vi"("error in (no error)"=w450, "Cluster"=w458) -> ("error out"=w452:errorcluster, "Array of VData"=w457:variant[])  [unwired: 8 in]
          n213 = for {
            tunnel: w457 -> [w465] mode=indexing
            tunnel: [w464] -> w456 mode=concatenating
            tunnel: [w463] -> w454 mode=indexing
            shift-right: [w461] -> w451
            shift-left: w452 -> [w462]
            tunnel: w449 -> [w460]
            tunnel: [w459] -> w448
            n214 = call "Mem_DataToU8Array.vi"("error in (no error)"=w462, "Payload"=w465, "AddrQueueIn"=w460) -> ("error out"=w461:errorcluster, "Supported Type?"=w463:bool, "ByteArray"=w464:u8[], "AddrQueueOut"=w459:refnum<queue>)  [unwired: 5 in]
          }
          n215 = Build Array (concatenate)(w456) -> (w455:u8[])
          n216 = And Array Elements(Boolean array=w454) -> (logical AND=w453:bool)
        }
      }
      "ByteArray" <- w10
      "Supported Type?" <- w9
      "AddrQueueOut" <- w4
    }
    frame Error {
    }
  }
  "error out" <- w2
